vi "Run Solver.vi"(7 "Words":string[](array[string]), 8 "error in":errorcluster, 10 "Scorer Context":refnum<vi>, 11 "Solver Ref":T1) -> (0 "error out":errorcluster, 2 "Success":bool, 3 "Avg Guesses":dbl=10.0, 4 "Min Guesses":i32, 6 "Max Guesses":i32)   [LabVIEW 2024, in "Wordle Scorer.lvlib"]
uses:
  Wordle Scorer.lvlib
  Solver VI Ref Type.ctl
  Libraries/Wordle Engine/Wordle Engine.lvlib
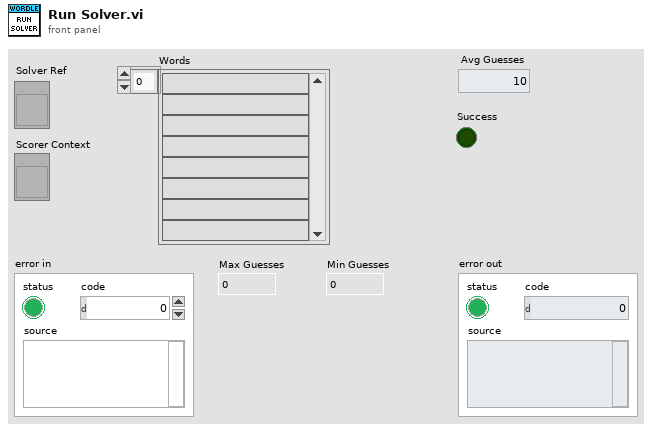
[diagram p1: front panel]
types:
  T1 = typedef "Wordle Scorer.lvlib/Solver VI Ref Type.ctl" = refnum<vi>
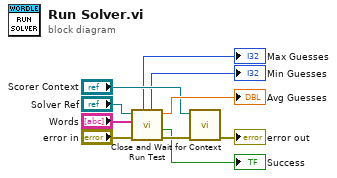
[diagram p0: block diagram]
diagram:
  n1 = call "Run Test.vi"("error in (no error)"="error in", "Words"="Words", "Solver Ref"="Solver Ref") -> ("error out"=w7:errorcluster, "Valid"=→"Success":bool, "Avg Guesses"=→"Avg Guesses":dbl, "Min Guesses"=→"Min Guesses":i32, "Max Guesses"=→"Max Guesses":i32)  [unwired: 3 in, 1 out]
  n2 = call "Close and Wait for Context.vi"("error in (no error)"=w7, "Scorer Context"="Scorer Context") -> ("error out"=→"error out":errorcluster)  [unwired: 9 in]
